vi "Maintenance_Modbus.vi"(0 "Modbus master in":refnum<class "Modbus Master.lvclass">, 2 "Modbus Inputs":T1, 5 "error in":errorcluster) -> (14 "Modbus master out":refnum<class "Modbus Master.lvclass">, 19 "error out":errorcluster)   [LabVIEW 2021]
uses:
  Controls/Modbus Input.ctl
  <vilib>/Modbus/master/Modbus Master.lvclass
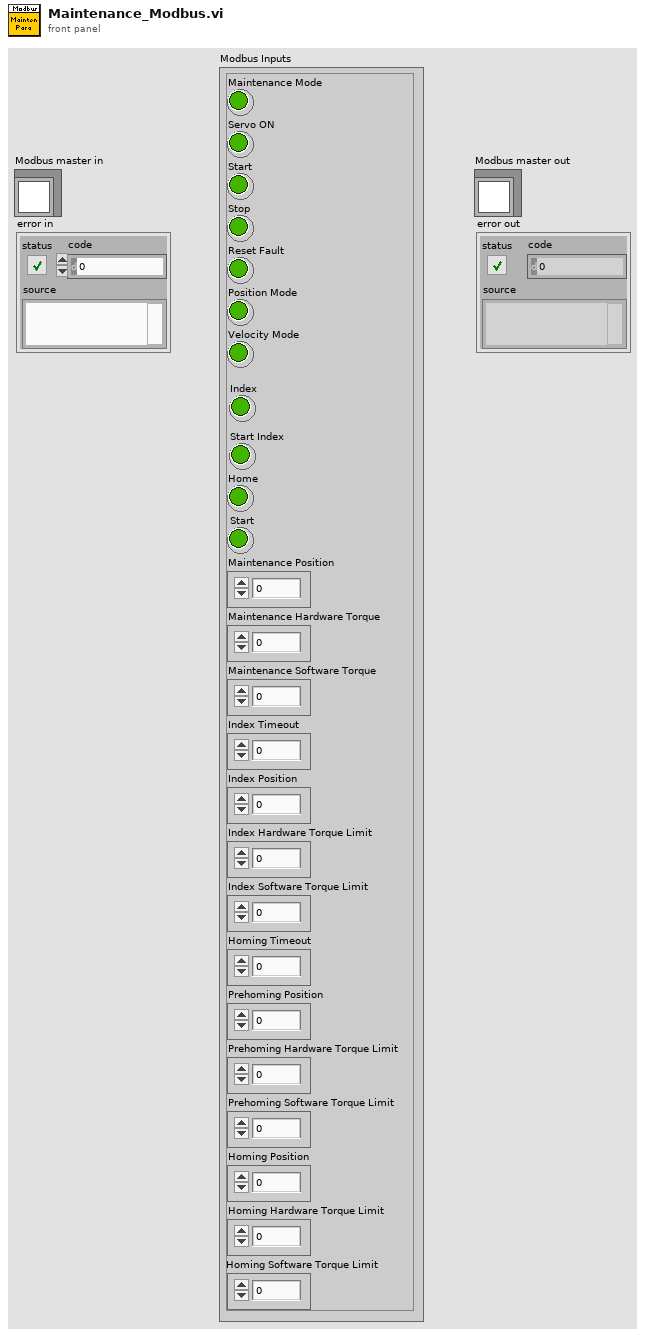
[diagram p1: front panel]
types:
  T1 = typedef "Modbus Input.ctl" = cluster{"Maintenance Mode":bool, "Servo ON":bool, "Start":bool, "Stop":bool, "Reset Fault":bool, "Position Mode":bool, "Velocity Mode":bool, "Index":bool, "Start Index":bool, "Home":bool, "Start":bool, "Maintenance Position":i32, "Maintenance Hardware Torque":u16, "Maintenance Software Torque":u16, "Index Timeout":i16, "Index Position":i32, "Index Hardware Torque Limit":u16, "Index Software Torque Limit":u16, "Homing Timeout":i16, "Prehoming Position":i32, "Prehoming Hardware Torque Limit":u16, "Prehoming Software Torque Limit":u16, "Homing Position":i32, "Homing Hardware Torque Limit":u16, "Homing Software Torque Limit":u16}
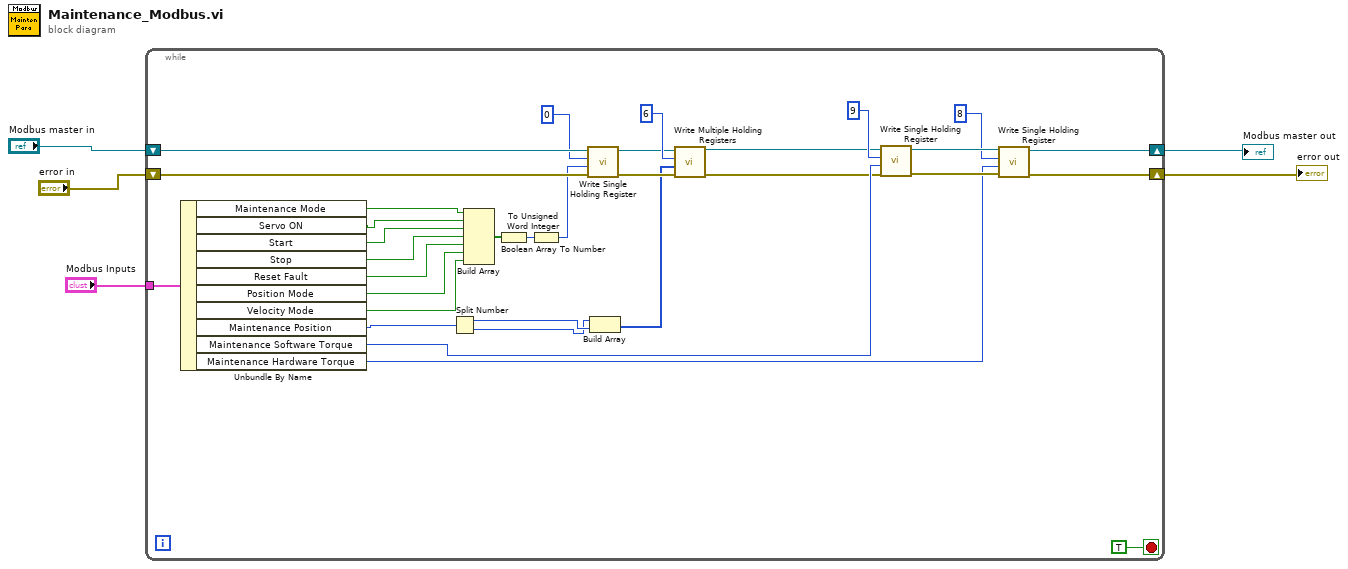
[diagram p0: block diagram]
diagram:
  n1 = while {
    shift-right: [w24] -> w5
    shift-left: "Modbus master in" -> [w37]
    shift-right: [w25] -> w4
    shift-left: "error in" -> [w36]
    tunnel: "Modbus Inputs" -> [w22]
    stop <- TRUE stop-if-true
    n2 = Unbundle By Name(w22) -> ("Maintenance Mode"=w21:bool, "Servo ON"=w11:bool, "Start"=w12:bool, "Stop"=w13:bool, "Reset Fault"=w14:bool, "Position Mode"=w20:bool, "Velocity Mode"=w19:bool, "Maintenance Position"=w17:i32, "Maintenance Software Torque"=w16:u16, "Maintenance Hardware Torque"=w15:u16)
    n3 = Split Number(x=w17) -> (hi(x)=w10:u16, lo(x)=w9:u16)
    n4 = Build Array(w21, w11, w12, w13, w14, w20, w19) -> (w18:bool[])
    n5 = Boolean Array To Number(Boolean array=w18) -> (number=w34:u32)
    n6 = To Unsigned Word Integer(number=w34) -> (unsigned 16bit integer=w33:u16)
    n7 = call-dynamic "Write Single Holding Register.vi"("error in (no error)"=w36, "holding register value"=w33, "address"=u16 0, "Modbus master in"=w37) -> ("error out"=w30:errorcluster, "Modbus master out"=w31:refnum<class "Modbus Master.lvclass">)  [unwired: 6 in]
    n8 = Build Array(w9, w10) -> (w8:u16[])
    n9 = call-dynamic "Write Multiple Holding Registers.vi"("error in (no error)"=w30, "holding register values"=w8, "starting address"=u16 6, "Modbus master in"=w31) -> ("error out"=w7:errorcluster, "Modbus master out"=w6:refnum<class "Modbus Master.lvclass">)  [unwired: 6 in]
    n10 = call-dynamic "Write Single Holding Register.vi"("error in (no error)"=w7, "holding register value"=w16, "address"=u16 9, "Modbus master in"=w6) -> ("error out"=w27:errorcluster, "Modbus master out"=w28:refnum<class "Modbus Master.lvclass">)  [unwired: 6 in]
    n11 = call-dynamic "Write Single Holding Register.vi"("error in (no error)"=w27, "holding register value"=w15, "address"=u16 8, "Modbus master in"=w28) -> ("error out"=w25:errorcluster, "Modbus master out"=w24:refnum<class "Modbus Master.lvclass">)  [unwired: 6 in]
  }
  "Modbus master out" <- w5
  "error out" <- w4
